vi "h.SYSTEM.GetInstrumentName.vi"(8 "error in":errorcluster, 11 "Connection ID In":refnum<k5>) -> (0 "error out":errorcluster, 2 "Instrument Name":string, 3 "Connection ID Out":refnum<k5>)   [LabVIEW 2016, in "h.Library.lvlib"]
doc: "Use this VI to retrieve the serial number of a Hyperion instrument.\n\n<b>Connection ID</b> - is a network connection refnum that uniquely identifies the TCP connection\n<b>Timeout</b> - specifies the maximum amount of time, in milliseconds, for the function to complete\n<b>error in</b> - describes error conditions that occur before this node runs. This input provides standard error functionality\n<b>Connection ID out</b> - returns the same value as connection ID\n<b>Serial Number</b> - serial number of the instrument\n<b>error out</b> - contains error information. This output provides standard error out functionality."
uses:
  h.Library.lvlib
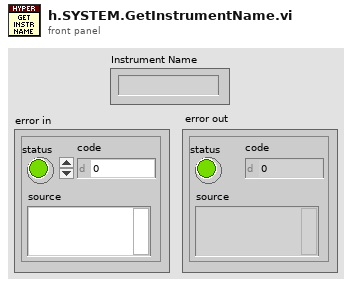
[diagram p1: front panel]
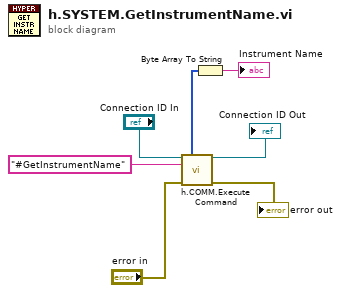
[diagram p0: block diagram]
diagram:
  n1 = call "h.COMM.Execute Command.vi"("Connection ID"="Connection ID In", "Command"="#GetInstrumentName", "error in"="error in") -> ("Content"=w4:u8[], "Connection ID out"=→"Connection ID Out":refnum<k5>, "error out"=→"error out":errorcluster)  [unwired: 5 in, 5 out]
  n2 = Byte Array To String(unsigned byte array=w4) -> (string=→"Instrument Name":string)
